vi "Periodic Tasks.vi"(8 "error in":errorcluster) -> ()   [LabVIEW 2014]
doc: "This VI runs in parallel to other tasks. It can contain as many user-defined periodic loops as you need. These can carry out PID or other sorts of timed response."
uses:
  Begin/Global RefNums.vi
panel:
  out "Elapsed Time (s)":dbl
  in  "Reset 2":bool caption="Reset"
  in  "Reset":bool
  out "Period (sec)":dbl
  out "Stopped":bool
  out "Direction":bool
  out "Value":i32
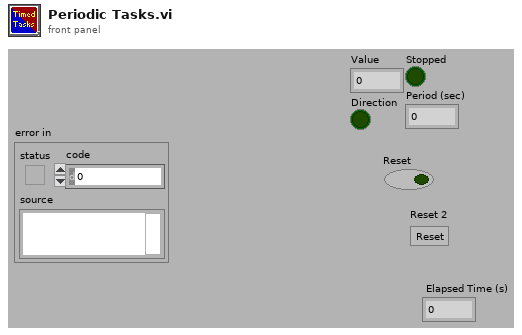
[diagram p1: front panel]
types:
  T1 = typedef "WPI_CounterDevRef.ctl" = cluster{"DevStatus":errorcluster, "CntIndex":T2}
  T2 = typedef "FPGA_CounterCtrSystemIndex.ctl" = enum8{"Ctr 0", "Ctr 1", "Ctr 2", "Ctr 3", "Ctr 4", "Ctr 5", "Ctr 6", "Ctr 7", "Invalid"}
  T3 = typedef "WPI_MotorControlDeviceRef.ctl" = cluster{"DeviceStatus":errorcluster, "Type":T4, "PWM":cluster{"Controller":T5, "PWM Channel":T6, "DeadBand":T7}, "CAN":cluster{"Device Number":u8, "Control Mode":T8, "Semaphore":T9, "Max Vout":dbl, "TalonSRX Control Mode":T10}, "Invert":bool, "TransformRef":T11, "InvTransformRef":T11}
  T4 = typedef "WPI_MotorControlType.ctl" = enum16{"PWM", "CAN", "CANTalonSRX"}
  T5 = typedef "FPGA_TypedefDigitalModule.ctl" = enum16{"Controller 1"}
  T6 = typedef "FPGA_DIOPWMChannel.ctl" = enum8{"PWM 0", "PWM 1", "PWM 2", "PWM 3", "PWM 4", "PWM 5", "PWM 6", "PWM 7", "PWM 8", "PWM 9", "PWM MXP 0", "PWM MXP 1", "PWM MXP 2", "PWM MXP 3", "PWM MXP 4", "PWM MXP 5", "PWM MXP 6", "PWM MXP 7", "PWM MXP 8", "PWM MXP 9", "Invalid"}
  T7 = typedef "WPI_PWMDeadband.ctl" = cluster{"Name":string, "maxPositivePwm":i32, "minPositivePwm":i32, "centerPwm":i32, "maxNegativePwm":i32, "minNegativePwm":i32, "angularRange":u16}
  T8 = typedef "WPI_CANJaguar_ControlMode.ctl" = enum8{"Percent VBus", "Current", "Speed", "Position", "Voltage"}
  T9 = typedef "Semaphore RefNum" = refnum<k1>
  T10 = typedef "WPI_CANTalonSRX_APIControlMode.ctl" = enum8{"Percent VBus", "Speed", "Position", "Slave", "Unchanged / Invalid"}
  T11 = typedef "WPI_PWMTransform_ConPane.ctl" = refnum<vi>
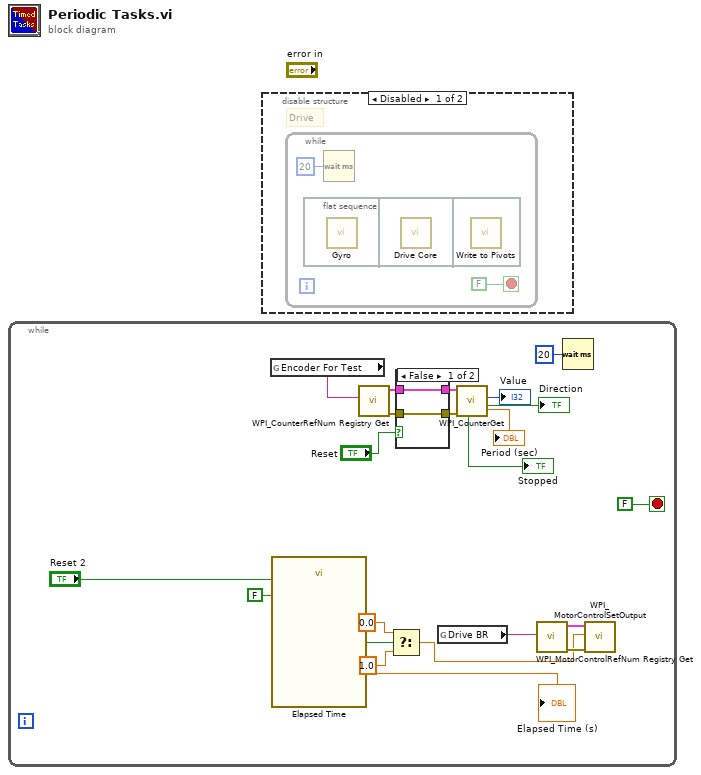
[diagram p0: block diagram]
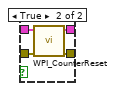
[diagram p3: hidden frame]
diagram:
  n1 = while {
    stop <- FALSE stop-if-true
    n2 = global read "Global RefNums.vi" "Encoder For Test"() -> (w22:string)
    n3 = call "Elapsed Time"("Reset"="Reset 2", "Auto Reset"=FALSE) -> ("Elapsed Time (s)"=→"Elapsed Time (s)":dbl, "Time has Elapsed"=w7:bool)  [unwired: 10 in, 6 out]
    n4 = call <vilib>:"WPI_CounterRefNum Registry Get.vi"("refnum name"=w22) -> ("error out"=w14:errorcluster, "CounterDevRef"=w16:T1)  [unwired: 9 in]
    n5 = Select(t=0.0, s=w7, f=1.0) -> (s? t:f=w4:dbl)
    n6 = case shown="False" "Reset" {
      tunnel: w16 -> [w24 w28]
      tunnel: [w24 w27] -> w15
      tunnel: w14 -> [w23 w26]
      tunnel: [w23 w25] -> w13
      frame False {
      }
      frame True {
        n7 = call <vilib>:"WPI_CounterReset.vi"("error in (no error)"=w26, "CounterDevRef in"=w28) -> ("error out"=w25:errorcluster, "CounterDevRef out"=w27:T1)  [unwired: 8 in]
      }
    }
    n8 = global read "Global RefNums.vi" "Drive BR"() -> (w10:string)
    n9 = call <vilib>:"WPI_CounterGet.vi"("error in (no error)"=w13, "CounterDevRef in"=w15) -> ("Direction"=→"Direction":bool, "Value"=→"Value":i32, "Period (sec)"=→"Period (sec)":dbl, "Stopped"=→"Stopped":bool)  [unwired: 4 in, 2 out]
    n10 = call <vilib>:"WPI_MotorControlRefNum Registry Get.vi"("refnum name"=w10) -> ("error out"=w9:errorcluster, "MotorControlDevRef"=w8:T3)  [unwired: 9 in]
    n11 = Wait (ms)(milliseconds to wait=u32 20) -> ()  [unwired: 1 out]
    n12 = call <vilib>:"WPI_MotorControlSetOutput.vi"("error in (no error)"=w9, "Output"=w4, "MotorControlDevRef"=w8) -> ()  [unwired: 6 in, 3 out]
  }
  n13 = disable-structure shown="Disabled" {
    frame Disabled {
      # "Drive"
      n14 = while {
        stop <- FALSE stop-if-true
        n15 = flat-sequence {
          frame #0 {
            n16 = call "Gyro.vi"() -> ()  [unwired: 12 in]
          }
          frame #1 {
            n17 = call "Drive Core.vi"() -> ()  [unwired: 12 in]
          }
          frame #2 {
            n18 = call "Write to Pivots.vi"() -> ()  [unwired: 12 in]
          }
        }
        n19 = Wait (ms)(milliseconds to wait=u32 20) -> ()  [unwired: 1 out]
      }
    }
    frame Enabled {
    }
  }
